vi "TDMS.GetAnalysisParameters.vi"(8 "error in (no error)":errorcluster, 11 "TDMS Ref":refnum<k34>) -> (0 "error out":errorcluster, 1 "Found?":bool, 2 "LVTransitionParameters":T1, 3 "TDMS Ref":refnum<k34>)   [LabVIEW 2015, in "TestStand Analysis Steps.lvlib"]
uses:
  TestStand Analysis Steps.lvlib
  Types/Public.LVAnalysis.ctl
  Types/Public.ChLVAnalysis.ctl
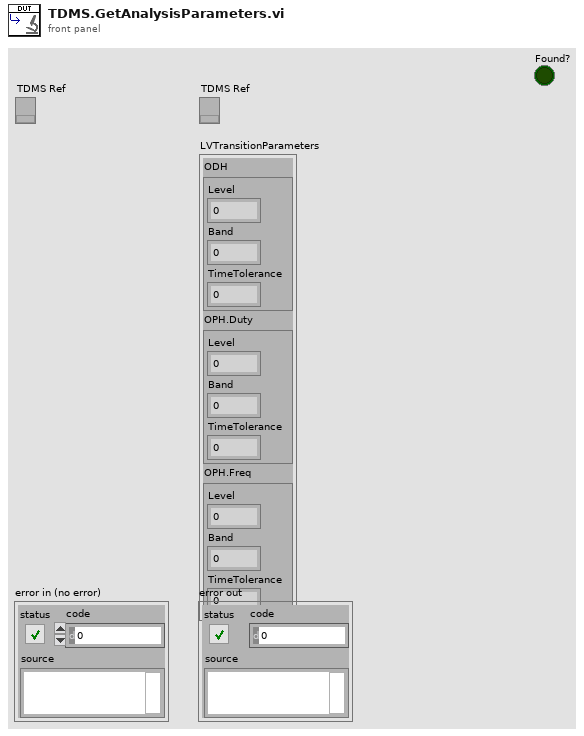
[diagram p1: front panel]
types:
  T1 = typedef "TestStand Analysis Steps.lvlib/Public.LVAnalysis.ctl" = cluster{"ODH":T2, "OPH.Duty":T2, "OPH.Freq":T2}
  T2 = typedef "TestStand Analysis Steps.lvlib/Public.ChLVAnalysis.ctl" = cluster{"Level":dbl, "Band":dbl, "TimeTolerance":dbl}
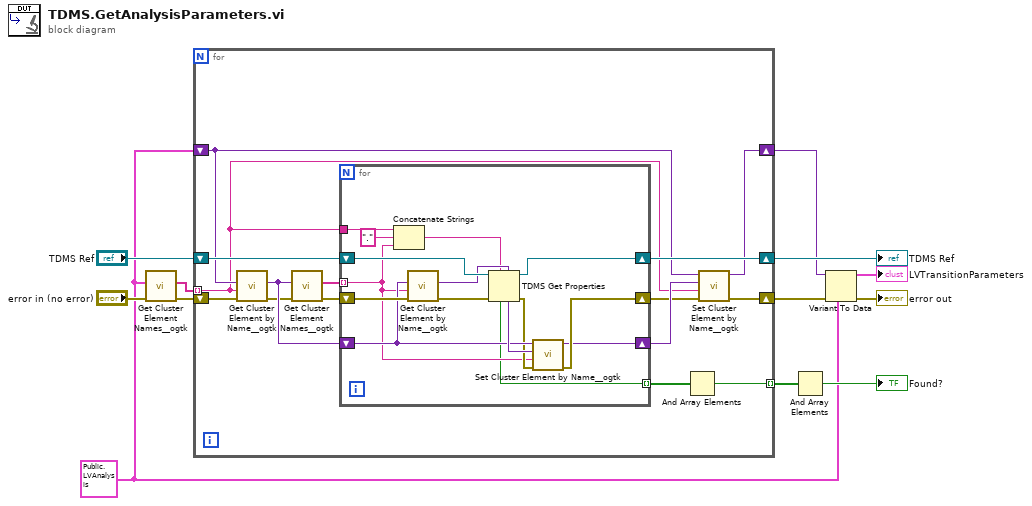
[diagram p0: block diagram]
diagram:
  w1 = T1 {"ODH"={"Level"=0.0, "Band"=0.0, "TimeTolerance"=0.0}, "OPH.Duty"={"Level"=0.0, "Band"=0.0, "TimeTolerance"=0.0}, "OPH.Freq"={"Level"=0.0, "Band"=0.0, "TimeTolerance"=0.0}} ("LVTransitionParameters")
  n1 = call <userlib>:"Get Cluster Element Names__ogtk.vi"("error in (no error)"="error in (no error)", "Cluster"=w1) -> ("error out"=w4:errorcluster, "Element Names"=w10:string[])  [unwired: 8 in]
  n2 = for {
    shift-right: [w18] -> w6
    shift-left: w4 -> [w25]
    shift-right: [w26] -> w8
    shift-left: "TDMS Ref" -> [w27]
    tunnel: w10 -> [w13] mode=indexing
    shift-right: [w17] -> w7
    shift-left: w1 -> [w16]
    tunnel: [w14] -> w5 mode=indexing
    n3 = call <userlib>:"Get Cluster Element by Name__ogtk.vi"("error in (no error)"=w25, "Element Name"=w13, "Cluster"=w16) -> ("error out"=w22:errorcluster, "VElement"=w24:variant)  [unwired: 6 in, 1 out]
    n4 = call <userlib>:"Get Cluster Element Names__ogtk.vi"("error in (no error)"=w22, "Cluster"=w24) -> ("error out"=w21:errorcluster, "Element Names"=w23:string[])  [unwired: 8 in]
    n5 = for {
      shift-right: [w41] -> w26
      shift-left: w27 -> [w42]
      shift-right: [w31] -> w19
      shift-left: w21 -> [w39]
      tunnel: w23 -> [w30] mode=indexing
      tunnel: w13 -> [w36]
      shift-right: [w29] -> w20
      shift-left: w24 -> [w33]
      tunnel: [w28] -> w15 mode=indexing
      n6 = Concatenate Strings(w36, "." ("string"), w30) -> (w35:string)
      n7 = call <userlib>:"Get Cluster Element by Name__ogtk.vi"("error in (no error)"=w39, "Element Name"=w30, "Cluster"=w33) -> ("error out"=w38:errorcluster, "VElement"=w40:variant)  [unwired: 6 in, 1 out]
      n8 = TDMS Get Properties(5:w40, 7:w35, 8:w38, 11:w42) -> (0:w32:errorcluster, 3:w41:refnum<k34>, 4:w34:variant, 6:w28:bool)  [unwired: 2 in, 2 out]
      n9 = call <userlib>:"Set Cluster Element by Name__ogtk.vi"("error in (no error)"=w32, "Element Name (\"\": New Element Data Name)"=w30, "New Element Value"=w34, "Cluster"=w33) -> ("error out"=w31:errorcluster, "VCluster out"=w29:variant)  [unwired: 5 in, 1 out]
    }
    n10 = And Array Elements(Boolean array=w15) -> (logical AND=w14:bool)
    n11 = call <userlib>:"Set Cluster Element by Name__ogtk.vi"("error in (no error)"=w19, "Element Name (\"\": New Element Data Name)"=w13, "New Element Value"=w20, "Cluster"=w16) -> ("error out"=w18:errorcluster, "VCluster out"=w17:variant)  [unwired: 5 in, 1 out]
  }
  "TDMS Ref" <- w8
  n12 = And Array Elements(Boolean array=w5) -> (logical AND=→"Found?":bool)
  n13 = Variant To Data(error in=w6, type=w1, Variant=w7) -> (data=→"LVTransitionParameters":T1, error out=→"error out":errorcluster)
